vi "PPMS_Measure.vi"(6 "error in (no error)":errorcluster, 7 "Index":i8) -> (0 "error out":errorcluster, 2 "resulting string 1":string="Measure Lockin Channe1, Channel2,  Averages 0 every 0 seconds", 3 "Cancelled?":bool=TRUE)   [LabVIEW 2017]
doc: "Use this template to create a dialog box. This template polls the state of the buttons on the front panel and does not use events. Use the Dialog Using Events template (not available in Base package) to create a dialog box with event handling."
panel:
  in  "#Time (SET MODE)":dbl=10.0
  in  "#Points (SCAN MODE)":u16=10
  out "MODE":i32(ring) items=["SET&MEAS", "SCAN", ""]
  in  "1 measure every (sec)":dbl=1.0 format="%.3f"
  in  "Averages":u16=10
  in  "Cancel":bool
  in  "OK":bool
  # "Octubre 2019 V1.2  a-sslcdms"
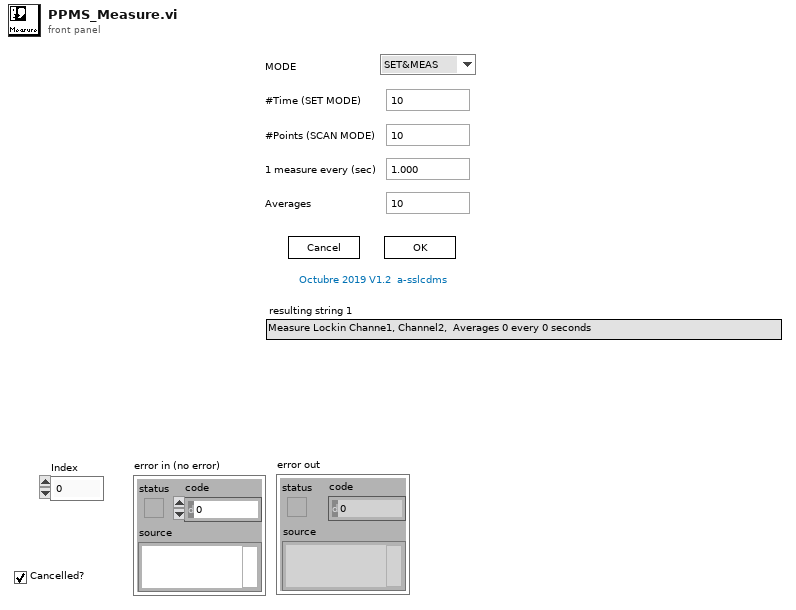
[diagram p1: front panel]
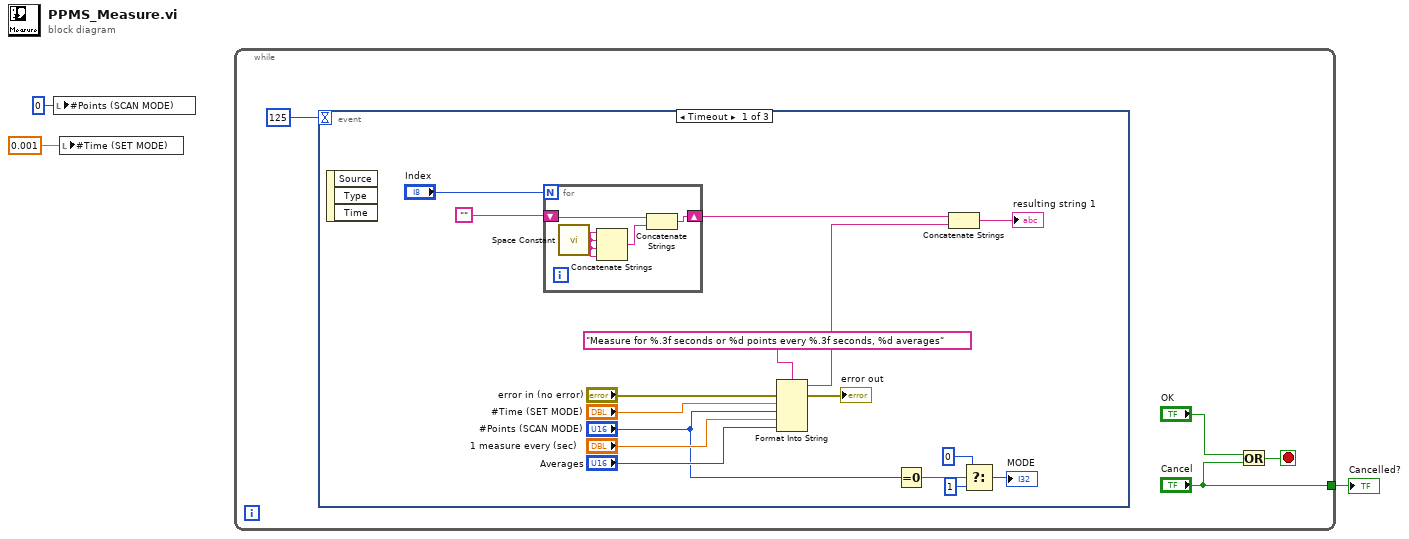
[diagram p0: block diagram]
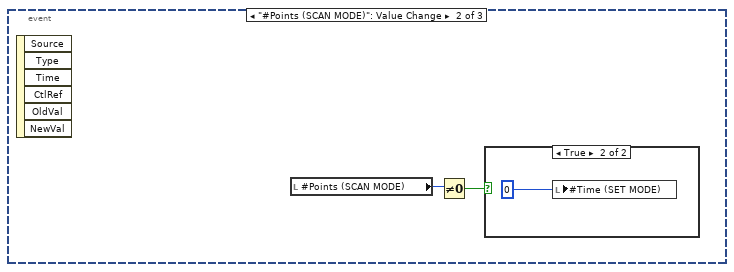
[diagram p2: hidden frame]
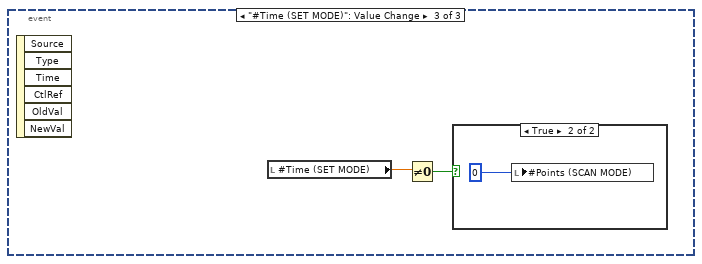
[diagram p4: hidden frame]
diagram:
  n1 = local write "#Points (SCAN MODE)"(u16 0 ("#Points (SCAN MODE)")) -> ()
  n2 = local write "#Time (SET MODE)"(0.001 ("#Points (SCAN MODE)")) -> ()
  n3 = while {
    tunnel: ["Cancel"] -> w3
    stop <- w6 stop-if-true
    n4 = event shown="[0] Timeout" {
      selector: _ -> [_ _ _]
      dyn-events: _ -> [_ _ _]
      timeout: 125 -> [_ _ _]
      event Timeout {
        n5 = event-data() -> ()  [unwired: 1 in, 3 out]
        n6 = for {
          N: "Index" -> [_]
          shift-right: [w26] -> w20
          shift-left: "" -> [w25]
          n7 = call <vilib>:"Space Constant.vi"() -> ("String"=w24:string)
          n8 = Concatenate Strings(w24, w24, w24, w24) -> (w27:string)
          n9 = Concatenate Strings(w25, w27) -> (w26:string)
        }
        n10 = Format Into String(format string="Measure for %.3f seconds or %d points every %.3f seconds, %d averages", error in="error in (no error)", "#Time (SET MODE)", "#Points (SCAN MODE)", "1 measure every (sec)", "Averages") -> (resulting string=w18:string, error out=→"error out":errorcluster)  [unwired: 1 in]
        n11 = Equal To 0?(x="#Points (SCAN MODE)") -> (x = 0?=w11:bool)
        n12 = Concatenate Strings(w20, w18) -> (→"resulting string 1":string)
        n13 = Select(t=0, s=w11, f=1) -> (s? t:f=→"MODE":i32)
      }
      event "#Points (SCAN MODE)": Value Change {
        n14 = event-data() -> ()  [unwired: 1 in, 6 out]
        n15 = local read "#Points (SCAN MODE)"() -> (w28:u16)
        n16 = Not Equal To 0?(x=w28) -> (x != 0?=w29:bool)
        n17 = case shown="True" w29 {
          frame False {
          }
          frame True {
            n18 = local write "#Time (SET MODE)"(u16 0 ("#Points (SCAN MODE)")) -> ()
          }
        }
      }
      event "#Time (SET MODE)": Value Change {
        n19 = event-data() -> ()  [unwired: 1 in, 6 out]
        n20 = local read "#Time (SET MODE)"() -> (w32:dbl)
        n21 = Not Equal To 0?(x=w32) -> (x != 0?=w31:bool)
        n22 = case shown="True" w31 {
          frame False {
          }
          frame True {
            n23 = local write "#Points (SCAN MODE)"(u16 0 ("#Points (SCAN MODE)")) -> ()
          }
        }
      }
    }
    n24 = Or(x="OK", y="Cancel") -> (x .or. y?=w6:bool)
  }
  "Cancelled?" <- w3
